vi "Get Harmonic Frequency.vi"(0 "Error In":errorcluster) -> (3 "Error Out":errorcluster, 4 "Show Ticks":bool, 5 "Harmonic frequency":dbl[unit])   [LabVIEW 2019]
uses:
  Phasor Explorer Settings List.ctl
  Phasor Explorer Phasor Parameters.ctl
  Phasor Calculation Type.ctl
  SEPL Type.ctl
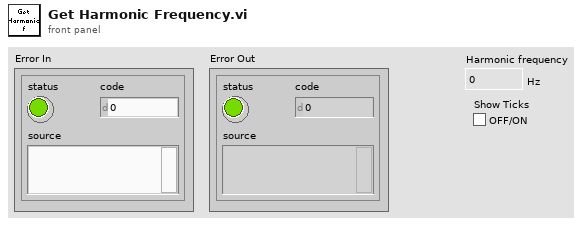
[diagram p1: front panel]
types:
  T1 = typedef "Phasor Explorer Phasor Parameters.ctl" = cluster{"Harmonic frequency":dbl[unit], "Use f* = 1/D Frequency":bool, "Calibrated Phasor":bool, "Calibration Lifetime":dbl[unit], "Phasor Calculation":T2, "SEPL Type":T3, "# Gates":dbl, "Square Gate Width":dbl[unit], "Show Ticks":bool}
  T2 = typedef "Phasor Calculation Type.ctl" = enum16{"Direct Sum", "Analytical Formula"}
  T3 = typedef "SEPL Type.ctl" = enum16{"UC", "L_N", "L_N[W]"}
  T4 = typedef "Phasor Explorer Settings List.ctl" = enum16{"Phasor Explorer Display Parameters", "Phasor Explorer Phasor Parameters", "Phasor Explorer Decay & IRF Parameters", "Phasor Explorer Gate Parameters", "Phasor Explorer Detector Parameters", "f*", "tau*"}
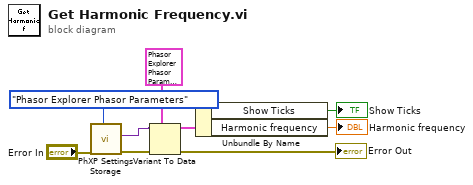
[diagram p0: block diagram]
diagram:
  n1 = call "PhXP Settings Storage.vi"("Error In"="Error In", "Settings List"=Phasor_Explorer_Settings_List."Phasor Explorer Phasor Parameters") -> ("Error Out"=w7:errorcluster, "Variant Data out"=w8:variant)  [unwired: 8 in]
  n2 = Variant To Data(error in=w7, type=T1 {"Harmonic frequency"=0.0, "Use f* = 1/D Frequency"=FALSE, "Calibrated Phasor"=FALSE, "Calibration Lifetime"=1e-09, "Phasor Calculation"=enum."Direct Sum", "SEPL Type"=enum."UC", "# Gates"=1.0, "Square Gate Width"=1e-09, "Show Ticks"=FALSE} ("Phasor Explorer Phasor Parameters"), Variant=w8) -> (data=w5:T1, error out=→"Error Out":errorcluster)
  n3 = Unbundle By Name(w5) -> ("Show Ticks"=→"Show Ticks":bool, "Harmonic frequency"=→"Harmonic frequency":dbl[unit])
